vi "LCAIO Get Out Chan Handle.vi"(8 "error in (no error)":errorcluster caption="Fehler (Eingang, kein Fehler)", 11 "Index":u8) -> (0 "error out":errorcluster caption="Fehler (Ausgang)", 3 "Analog Output Channel":i64)   [LabVIEW 2021, in "labbCAN_AnalogIO_API.lvlib"]
doc: "LCAIO_Func long LCAIO_CALL LCAIO_GetOutChanHandle(unsigned char Index,\n dev_hdl* pOutChanHdl);"
uses:
  labbCAN_AnalogIO_API.lvlib
  labbCAN_AnalogIO_API.dll
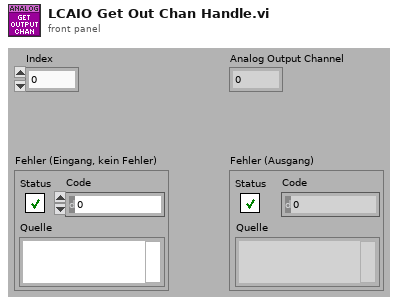
[diagram p1: front panel]
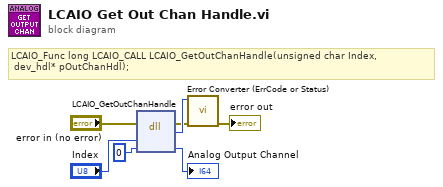
[diagram p0: block diagram]
diagram:
  # "LCAIO_Func long LCAIO_CALL LCAIO_GetOutChanHandle(unsigned char Index,\n\tdev_hdl* pOutChanHdl);"
  n1 = dll-call lib="C:/Users/olaja/AppData/Local/CETONI_SDK/labbCAN_AnalogIO_API.*" fn="LCAIO_GetOutChanHandle"(error in="error in (no error)", "Index"="Index", "pOutChanHdl"=i64 0) -> (error out=w2:errorcluster, "Rückgabetyp"=w3:i32, "pOutChanHdl"=→"Analog Output Channel":i64)  [unwired: 3 in, 1 out]
  n2 = call "Error Converter (ErrCode or Status).vi"("error in (no error)"=w2, "error code"=w3) -> ("error out"=→"error out":errorcluster)  [unwired: 9 in]
